vi "Replace XML Node.vi"(2 "error in (no error)":errorcluster, 3 "New node value":string="OK", 4 "Node name":string="Sample", 5 "XML String in":string="<?xml version=\"1.0\" encoding=\"utf-8\"?>\n<TestStructure>\n  <example>\n  <Sample>0</Sample>\n  <Sample>0</Sample>\n  </example>\n</TestStructure>") -> (0 "error out":errorcluster, 1 "XML String out":string)   [LabVIEW 2016]
uses:
  <vilib>/xml/Close Reference(Node).vi
  <vilib>/xml/NI_XML.lvlib
  <resource>/objmgr/DOMUserDefRef.rc
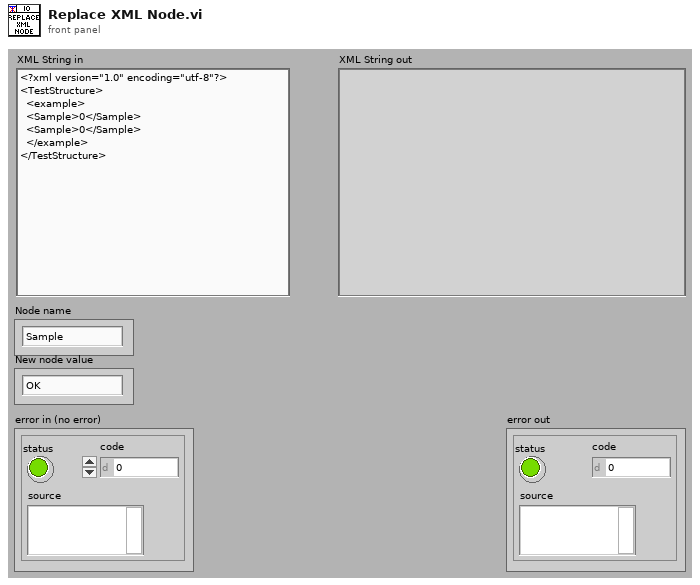
[diagram p1: front panel]
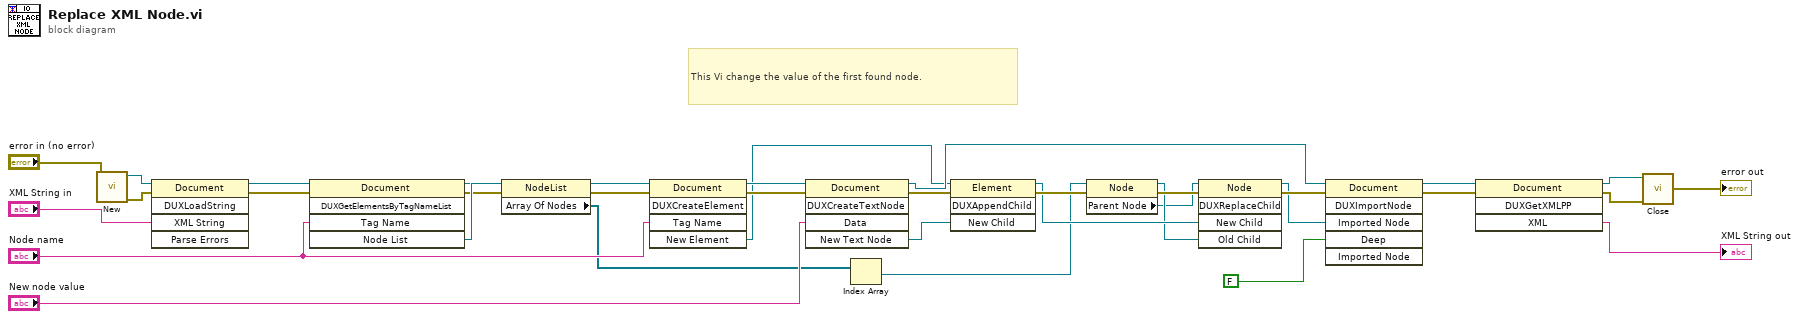
[diagram p0: block diagram]
diagram:
  # "This Vi change the value of the first found node."
  n1 = call <vilib>:"New.vi"("error in (no error)"="error in (no error)") -> ("error out"=w31:errorcluster, "DOM document out"=w32:refnum<k20>)  [unwired: 7 out]
  n2 = invoke class="Document" method="DUXLoadString"(reference=w32, error in=w31, "XML String"="XML String in") -> (reference out=w29:refnum<k20>, error out=w30:errorcluster)  [unwired: 2 in, 3 out]
  n3 = invoke class="Document" method="DUXGetElementsByTagNameList"(reference=w29, error in=w30, "Tag Name"="Node name") -> (reference out=w4:refnum<k20>, error out=w22:errorcluster, "Node List"=w28:refnum<k20>)  [unwired: 2 in, 2 out]
  n4 = property class="NodeList"(reference=w28, error in=w22) -> (error out=w21:errorcluster, "Array Of Nodes"=w16:refnum<k20>[])  [unwired: 1 out]
  n5 = invoke class="Document" method="DUXCreateElement"(reference=w4, error in=w21, "Tag Name"="Node name") -> (reference out=w26:refnum<k20>, error out=w27:errorcluster, "New Element"=w15:refnum<k20>)  [unwired: 2 in, 2 out]
  n6 = invoke class="Document" method="DUXCreateTextNode"(reference=w26, error in=w27, "Data"="New node value") -> (reference out=w20:refnum<k20>, error out=w24:errorcluster, "New Text Node"=w14:refnum<k20>)  [unwired: 2 in, 2 out]
  n7 = Index Array(array=w16) -> (element=w3:refnum<k20>)  [unwired: 1 in]
  n8 = invoke class="Element" method="DUXAppendChild"(reference=w15, error in=w24, "New Child"=w14) -> (reference out=w13:refnum<k20>, error out=w23:errorcluster)  [unwired: 1 in, 2 out]
  n9 = property class="Node"(reference=w3, error in=w23) -> (reference out=w11:refnum<k20>, error out=w12:errorcluster, "Parent Node"=w9:refnum<k20>)
  n10 = invoke class="Node" method="DUXReplaceChild"(reference=w9, error in=w12, "New Child"=w13, "Old Child"=w11) -> (reference out=w8:refnum<k20>, error out=w10:errorcluster)  [unwired: 1 in, 3 out]
  n11 = invoke class="Document" method="DUXImportNode"(reference=w20, error in=w10, "Imported Node"=w8, "Deep"=FALSE) -> (reference out=w19:refnum<k20>, error out=w17:errorcluster)  [unwired: 2 in, 4 out]
  n12 = invoke class="Document" method="DUXGetXMLPP"(reference=w19, error in=w17) -> (reference out=w5:refnum<k20>, error out=w6:errorcluster, "XML"=→"XML String out":string)  [unwired: 2 in, 1 out]
  n13 = call-poly <vilib>:"Close.vi"("error in (no error)"=w6, "node"=w5) -> ("error out"=→"error out":errorcluster)  [unwired: 7 in]
